vi "Продукты 22.vi"() -> ()   [LabVIEW 2020]
uses:
  Control 11.ctl
panel:
  out "Корзина":T1[](array[typedef]) {"Температура С*" scale=0.0..100.0; "Годен до" format="%<%2d/%2m/%4Y>T"; "Дата изготовления" format="%<%2d/%2m/%4Y>T"}
  out "Сегодня":timestamp format="%<%2d/%2m/%4Y>T"
  out "Корзина":string
  in  "Удалить":bool
  out "База":T1[](array[typedef]) {"Температура С*" scale=0.0..100.0; "Годен до" format="%<%2d/%2m/%4Y>T"; "Дата изготовления" format="%<%2d/%2m/%4Y>T"}
  in  "stop":bool
  out "String":string
  in  "Добавить":bool
  in  "Добавляемый \nпродукт":T2 {"Температура С*" scale=0.0..100.0; "Годен до" format="%<%2d/%2m/%4Y>T"; "Дата изготовления" format="%<%2d/%2m/%4Y>T"}
  in  "Удаляемый продукт":T1 {"Температура С*" scale=0.0..100.0; "Годен до" format="%<%2d/%2m/%4Y>T"; "Дата изготовления" format="%<%2d/%2m/%4Y>T"}
  # "Добавить"
  # "Купить"
  # "Условия хранения"
  # "%"
  # "Пищевая ценность"
  # "Условия хранения"
  # "%"
  # "Пищевая ценность"
  # "Условия хранения"
  # "%"
  # "Пищевая ценность"
  # "Условия хранения"
  # "%"
  # "Пищевая ценность"
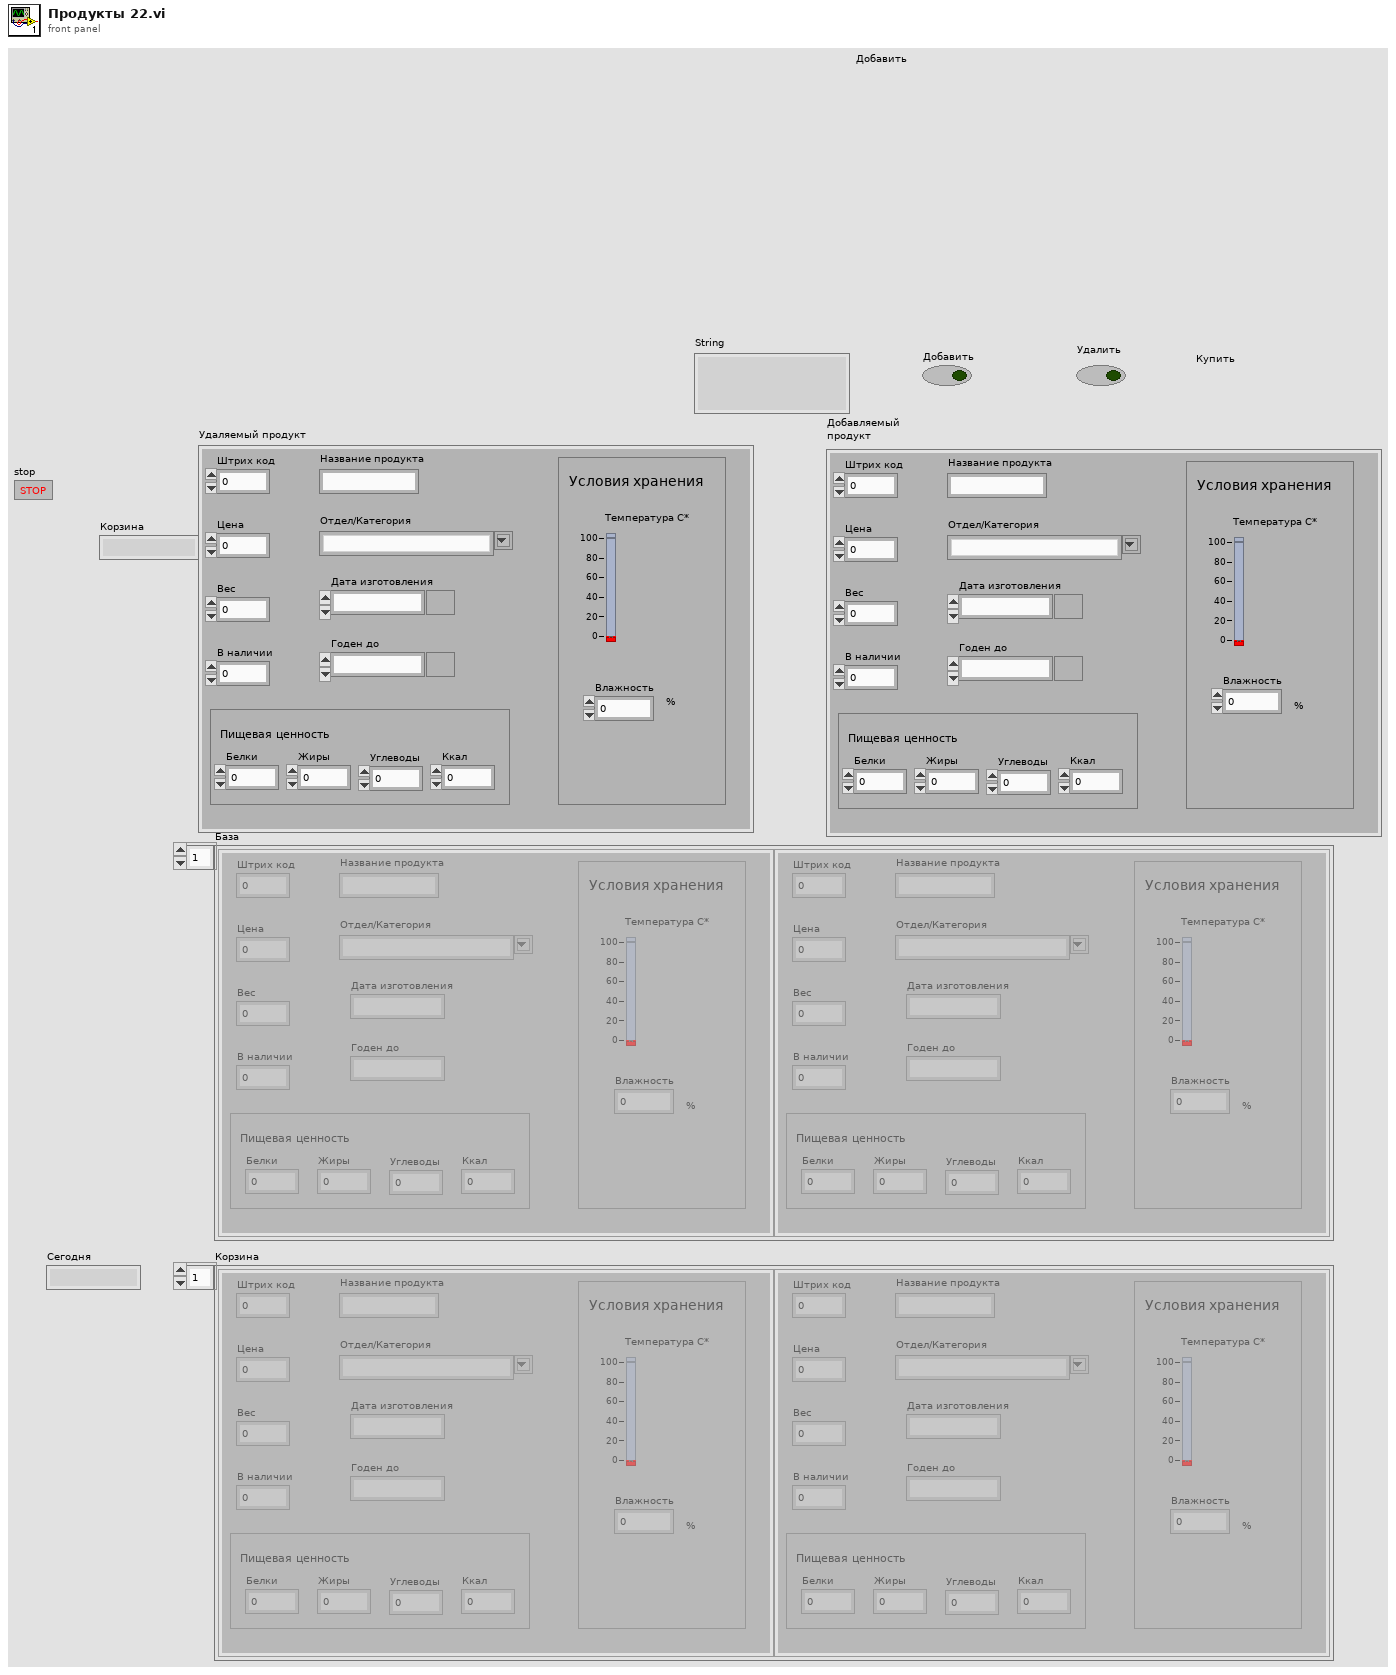
[diagram p1: front panel]
types:
  T1 = typedef "Control 11.ctl" = cluster{"Штрих код":dbl, "Цена":dbl, "Вес":dbl, "В наличии":dbl, "Дата изготовления":timestamp, "Годен до":timestamp, "Название продукта":string, "Температура С*":dbl, "Отдел/Категория":string, "Белки":dbl, "Жиры":dbl, "Углеводы":dbl, "Ккал":dbl, "Влажность":dbl}
  T2 = cluster{"Штрих код":dbl, "Цена":dbl, "Вес":dbl, "В наличии":dbl, "Дата изготовления":timestamp, "Годен до":timestamp, "Название продукта":string, "Температура С*":dbl, "Отдел/Категория":string, "Белки":dbl, "Жиры":dbl, "Углеводы":dbl, "Ккал":dbl, "Влажность":dbl}
  T3 = typedef "LVDateTimeRec.ctl" = cluster{"fractional second":dbl, "second":i32, "minute":i32, "hour":i32, "day of month":i32, "month":i32, "year":i32, "day of week":i32, "day of year":i32, "DST":i32}
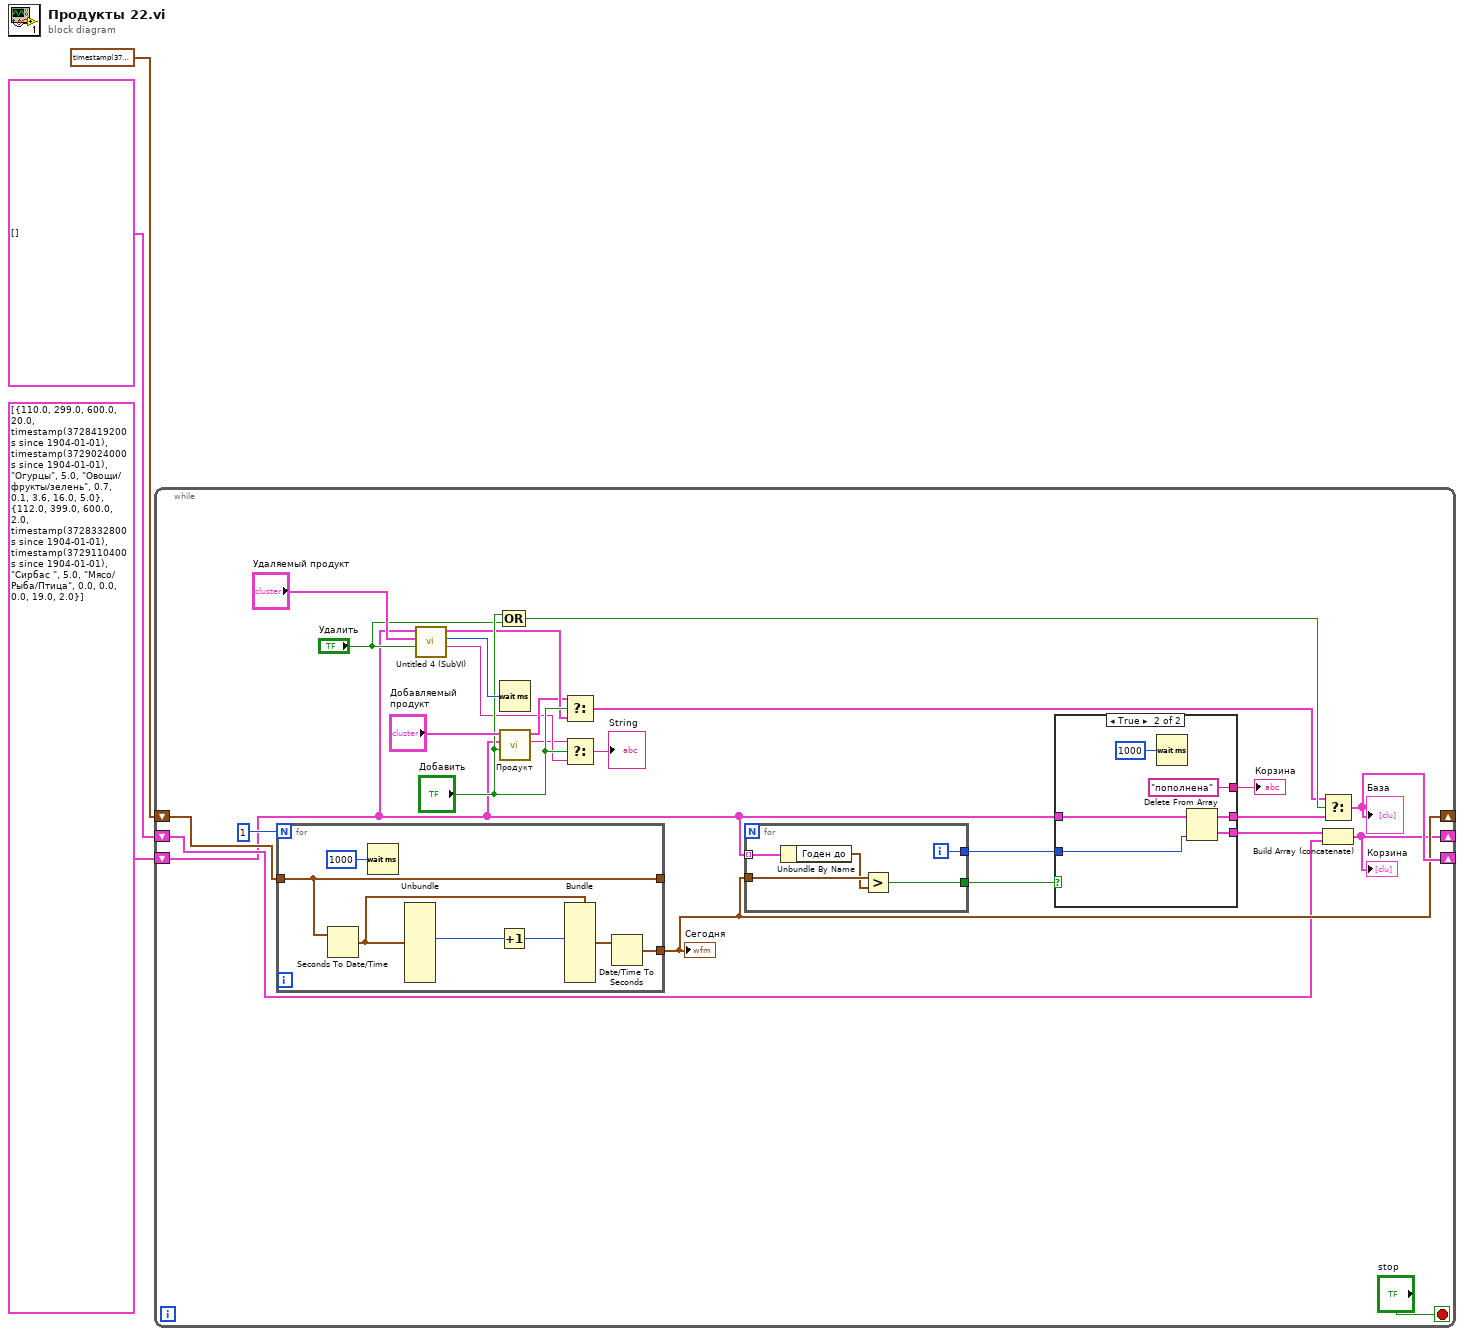
[diagram p0: block diagram]
diagram:
  n1 = while {
    shift-right: [w21] -> _
    shift-left: T1[] [{"Штрих код"=110.0, "Цена"=299.0, "Вес"=600.0, "В наличии"=20.0, "Дата изготовления"=timestamp(3728419200 s since 1904-01-01), "Годен до"=timestamp(3729024000 s since 1904-01-01), "Название продукта"="Огурцы", "Температура С*"=5.0, "Отдел/Категория"="Овощи/фрукты/зелень", "Белки"=0.7, "Жиры"=0.1, "Углеводы"=3.6, "Ккал"=16.0, "Влажность"=5.0}, {"Штрих код"=112.0, "Цена"=399.0, "Вес"=600.0, "В наличии"=2.0, "Дата изготовления"=timestamp(3728332800 s since 1904-01-01), "Годен до"=timestamp(3729110400 s since 1904-01-01), "Название продукта"="Сирбас ", "Температура С*"=5.0, "Отдел/Категория"="Мясо/Рыба/Птица", "Белки"=0.0, "Жиры"=0.0, "Углеводы"=0.0, "Ккал"=19.0, "Влажность"=2.0}] -> [w4]
    shift-right: [w9] -> _
    shift-left: timestamp(3729531600 s since 1904-01-01) -> [w10]
    shift-right: [w5] -> _
    shift-left: T1[] [] -> [w6]
    stop <- "stop" stop-if-true
    n2 = for {
      N: 1 -> [_]
      tunnel: [w43] -> w9
      tunnel: [w42] -> _
      tunnel: w10 -> [w42]
      n3 = Seconds To Date/Time(time stamp (now)=w42) -> (date time rec=w45:T3)  [unwired: 1 in]
      n4 = Wait (ms)(milliseconds to wait=u32 1000) -> ()  [unwired: 1 out]
      n5 = Unbundle(w45) -> ("day of month"=w44:i32)  [unwired: 9 out]
      n6 = Increment(x=w44) -> (x+1=w47:i32)
      n7 = Bundle(cluster=w45, "day of month"=w47) -> (w46:T3)  [unwired: 9 in]
      n8 = Date/Time To Seconds(2:w46) -> (0:w43:timestamp)  [unwired: 1 in]
    }
    "Сегодня" <- w9
    n9 = call "Untitled 4 (SubVI).vi"("Удалить"="Удалить", "Удаляемый продукт"="Удаляемый продукт", "Array in"=w4) -> ("String"=w17:string, "milliseconds to wait"=w26:u32, "Array out"=w20:T1[])  [unwired: 6 in]
    n10 = Wait (ms)(milliseconds to wait=w26) -> ()  [unwired: 1 out]
    n11 = call "Продукт"("Добавить"="Добавить", "Array in"=w4, "Добавляемый \nпродукт"="Добавляемый \nпродукт") -> ("String"=w16:string, "Array out"=w19:T1[])  [unwired: 7 in]
    n12 = Compound Arithmetic op=OR("Добавить", "Удалить") -> (w22:bool)
    n13 = Select(t=w19, s="Добавить", f=w20) -> (s? t:f=w18:T1[])
    n14 = Select(t=w16, s="Добавить", f=w17) -> (s? t:f=→"String":string)
    n15 = for {
      tunnel: [w33] -> w13
      tunnel: [w32] -> w14
      tunnel: w4 -> [w31] mode=indexing
      tunnel: w9 -> [w30]
      i -> [w32]
      n16 = Unbundle By Name(w31) -> ("Годен до"=w29:timestamp)
      n17 = Greater?(x=w30, y=w29) -> (0:w33:bool)
    }
    n18 = case shown="True" w13 {
      tunnel: [_ "пополнена"] -> w11
      tunnel: [_ w39] -> w7
      tunnel: w14 -> [_ w38]
      tunnel: w4 -> [w34 w37]
      tunnel: [w34 w36] -> w12
      frame False {
      }
      frame True {
        n19 = Wait (ms)(milliseconds to wait=u32 1000) -> ()  [unwired: 1 out]
        n20 = Delete From Array(array=w37, index=w38) -> (deleted portion=w39:T1, array with subset deleted=w36:T1[])  [unwired: 1 in]
      }
    }
    "Корзина" <- w11
    n21 = Select(t=w18, s=w22, f=w12) -> (s? t:f=w21:T1[])
    "База" <- w21
    n22 = Build Array (concatenate)(w7, w6) -> (w5:T1[])
    "Корзина" <- w5
  }
